vi "FTW-Container-New-FromContainer.vi"(5 "Container":variant, 11 "error in":errorcluster) -> (4 "FTW-Container":refnum<class "FTW-Container.lvclass">, 15 "error out":errorcluster)   [LabVIEW 2015, in "FTW-Container.lvclass"]
uses:
  FTW-Container.lvclass
  FTW-Container.lvclass/FTW-Container.ctl
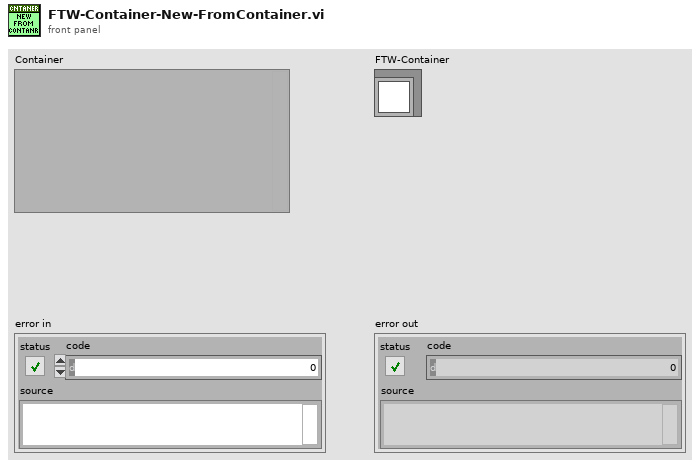
[diagram p1: front panel]
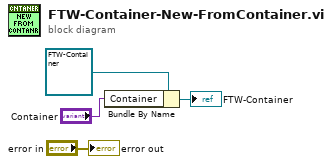
[diagram p0: block diagram]
diagram:
  n1 = Bundle By Name(cluster=refnum<class "FTW-Container.lvclass"> refnum ("FTW-Container"), "Container"="Container") -> (→"FTW-Container":refnum<class "FTW-Container.lvclass">)
  "error out" <- "error in"
